vi "Calc dependand variables.vi"(11 "Item Names":string[][](array[string])) -> (3 "Dependand Variables":T1)   [LabVIEW 2025]
uses:
  Controls/Dependand_Variables.ctl
  <vilib>/Analysis/baseanly.llb/Mean (DBL).vi
  <vilib>/regexp/Match Regular Expression.xnode
  <vilib>/Analysis/NI_AALBase.lvlib
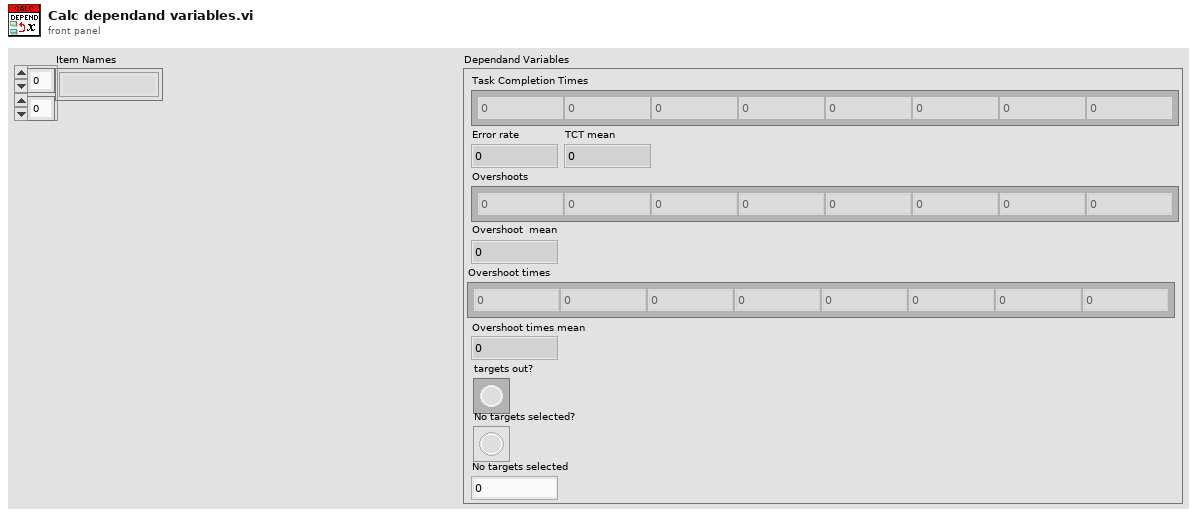
[diagram p1: front panel]
types:
  T1 = typedef "Dependand_Variables.ctl" = cluster{"Task Completion Times":dbl[], "TCT mean":dbl, "Error rate":i32, "Overshoots":i32[], "Overshoot  mean":dbl, "Overshoot times":dbl[], "Overshoot times mean":dbl, "targets out?":bool[], "No targets selected?":bool[], "No targets selected":i32}
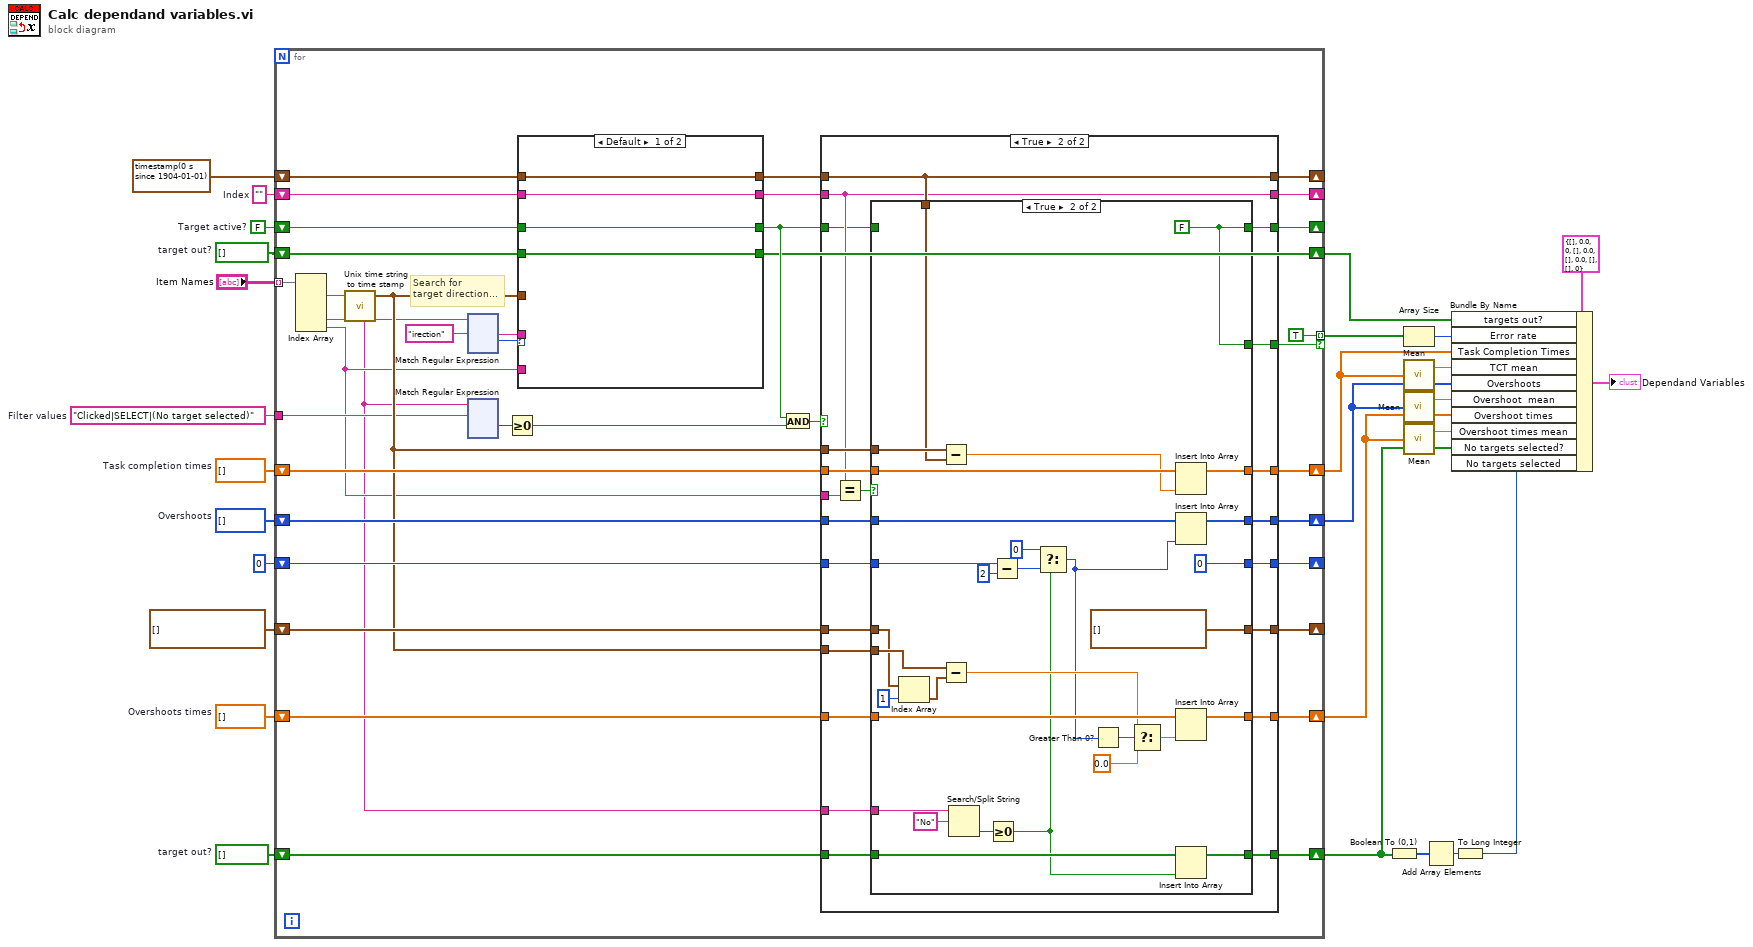
[diagram p0: block diagram]
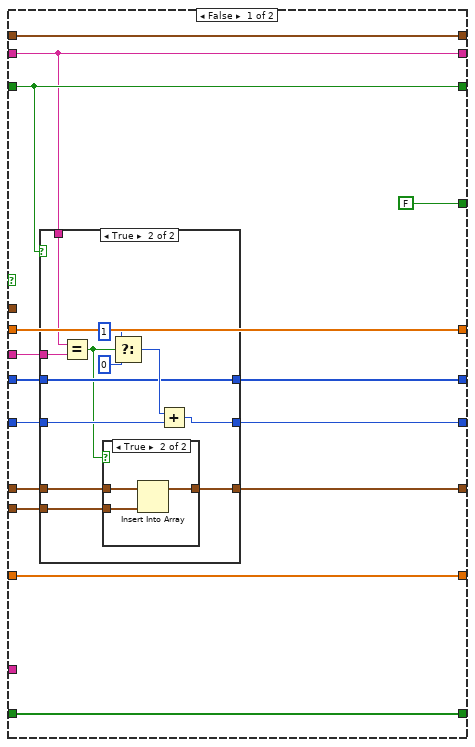
[diagram p2: hidden frame]
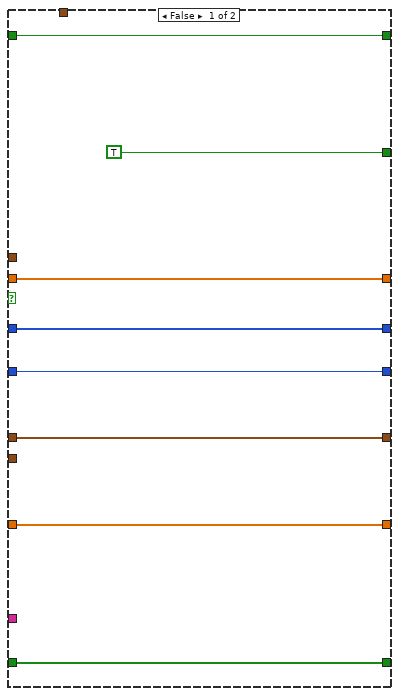
[diagram p5: hidden frame]
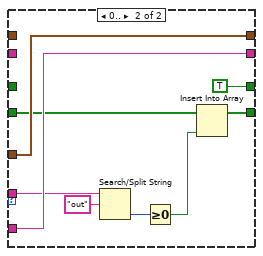
[diagram p6: hidden frame]
diagram:
  w5 = bool[] []  # target out?
  w7 = bool[] []  # target out?
  w18 = "Clicked|SELECT|(No target selected)"  # Filter values
  w27 = dbl[] []  # Overshoots times
  w24 = i32[] []  # Overshoots
  w23 = dbl[] []  # Task completion times
  w22 = FALSE  # Target active?
  w21 = ""  # Index
  n1 = for {
    tunnel: "Item Names" -> [w64] mode=indexing
    shift-right: [w57] -> _
    shift-left: timestamp(0 s since 1904-01-01) ("Time stamp") -> [w61]
    shift-right: [w56] -> _
    shift-left: w21 -> [w60]
    shift-right: [w54] -> _
    shift-left: w22 -> [w59]
    shift-right: [w52] -> w13
    shift-left: w23 -> [w53]
    tunnel: [TRUE] -> w16 mode=indexing if=w48
    shift-right: [w45] -> w11
    shift-left: w24 -> [w46]
    shift-right: [w43] -> _
    shift-left: 0 -> [w44]
    shift-right: [w40] -> _
    shift-left: timestamp[] [] -> [w42]
    shift-right: [w38] -> w9
    shift-left: w27 -> [w39]
    tunnel: w18 -> [w37]
    shift-right: [w34] -> w6
    shift-left: w7 -> [w33]
    shift-right: [w30] -> w4
    shift-left: w5 -> [w31]
    # "Search for\ntarget direction..."
    n2 = Index Array(array=w64) -> (element #1=w63:string, element #4=w28:string, element #5=w29:string)  [unwired: 5 in, 2 out]
    n3 = call "Unix time string to time stamp.vi"("Unix time string [ms]"=w63) -> ("Time stamp"=w41:timestamp)  [unwired: 4 in]
    n4 = xnode "Match Regular Expression"("input string"=w28, "regular expression"="irection" ("search string/char (-)")) -> ("after match"=w35:string, "offset past match"=w62:i32)  [unwired: 4 in, 3 out]
    n5 = xnode "Match Regular Expression"("input string"=w28, "regular expression"=w37) -> ("offset past match"=w47:i32)  [unwired: 4 in, 4 out]
    n6 = Greater Or Equal To 0?(x=w47) -> (x >= 0?=w32:bool)
    n7 = case shown="Default" w62 {
      tunnel: w41 -> [_ w406]
      tunnel: [w397 w406] -> w58
      tunnel: w61 -> [w397 _]
      tunnel: w29 -> [_ w405]
      tunnel: [w396 w405] -> w55
      tunnel: w60 -> [w396 _]
      tunnel: w59 -> [w395 _]
      tunnel: [w395 TRUE] -> w50
      tunnel: w35 -> [_ w403]
      tunnel: [w394 w399] -> w34
      tunnel: w33 -> [w394 w400]
      frame Default {
      }
      frame 0.. {
        n8 = Search/Split String(string=w403, search string/char (-)="out") -> (offset of match=w401:i32)  [unwired: 1 in, 2 out]
        n9 = Greater Or Equal To 0?(x=w401) -> (x >= 0?=w398:bool)
        n10 = Insert Into Array(array=w400, new element=w398) -> (w399:bool[])  [unwired: 1 in]
      }
    }
    n11 = And(x=w50, y=w32) -> (x .and. y?=w51:bool)
    n12 = case shown="True" w51 {
      tunnel: w41 -> [_ w353]
      tunnel: w58 -> [w313 w352]
      tunnel: [w313 w352] -> w57
      tunnel: [w308 w348] -> w56
      tunnel: w55 -> [w308 w348]
      tunnel: w50 -> [w310 w346]
      tunnel: [w310 w354] -> w54
      tunnel: w53 -> [w312 w351]
      tunnel: [w312 w350] -> w52
      tunnel: w29 -> [w309 w349]
      tunnel: [FALSE w345] -> w48
      tunnel: w46 -> [w304 w344]
      tunnel: [w305 w343] -> w45
      tunnel: w44 -> [w307 w342]
      tunnel: [w306 w341] -> w43
      tunnel: w42 -> [w303 w340]
      tunnel: w41 -> [w302 w338]
      tunnel: [w301 w339] -> w40
      tunnel: [w300 w337] -> w38
      tunnel: w39 -> [w300 w336]
      tunnel: w31 -> [w299 w335]
      tunnel: [w299 w334] -> w30
      tunnel: w28 -> [_ w333]
      frame False {
        n13 = case shown="True" w310 {
          tunnel: w309 -> [_ w328]
          tunnel: w308 -> [_ w327]
          tunnel: w307 -> [w316 w324]
          tunnel: [w316 w322] -> w306
          tunnel: [w315 w321] -> w305
          tunnel: w304 -> [w315 w321]
          tunnel: w303 -> [w314 w319]
          tunnel: w302 -> [_ w318]
          tunnel: [w314 w317] -> w301
          frame False {
          }
          frame True {
            n14 = Equal?(x=w327, y=w328) -> (x = y?=w320:bool)
            n15 = case shown="True" w320 {
              tunnel: w319 -> [w329 w332]
              tunnel: w318 -> [_ w331]
              tunnel: [w329 w330] -> w317
              frame False {
              }
              frame True {
                n16 = Insert Into Array(array=w332, new element=w331) -> (w330:timestamp[])  [unwired: 1 in]
              }
            }
            n17 = Select(t=1, s=w320, f=0 ("t")) -> (s? t:f=w323:i32)
            n18 = Add(x=w323, y=w324) -> (x+y=w322:i32)
          }
        }
      }
      frame True {
        n19 = Equal?(x=w348, y=w349) -> (x = y?=w347:bool)
        n20 = case shown="True" w347 {
          tunnel: [w362 w388] -> w354
          tunnel: w353 -> [_ w393]
          tunnel: w352 -> [_ w392]
          tunnel: w351 -> [w361 w391]
          tunnel: [w361 w389] -> w350
          tunnel: w346 -> [w362 _]
          tunnel: [TRUE w388] -> w345
          tunnel: w344 -> [w359 w387]
          tunnel: [w359 w386] -> w343
          tunnel: w342 -> [w358 w384]
          tunnel: [w358 0] -> w341
          tunnel: w340 -> [w356 w380]
          tunnel: [w356 timestamp[] []] -> w339
          tunnel: w338 -> [_ w381]
          tunnel: [w357 w377] -> w337
          tunnel: w336 -> [w357 w378]
          tunnel: w335 -> [w355 w371]
          tunnel: [w355 w370] -> w334
          tunnel: w333 -> [_ w367]
          frame False {
          }
          frame True {
            w388 = FALSE
            n21 = Index Array(array=w380, index=1) -> (element=w379:timestamp)
            n22 = Subtract(x=w393, y=w392) -> (x-y=w390:dbl)
            n23 = Subtract(x=w381, y=w379) -> (x-y=w374:dbl)
            n24 = Search/Split String(string=w367, search string/char (-)="No") -> (offset of match=w369:i32)  [unwired: 1 in, 2 out]
            n25 = Greater Or Equal To 0?(x=w369) -> (x >= 0?=w363:bool)
            n26 = Subtract(x=w384, y=2) -> (x-y=w366:i32)
            n27 = Select(t=0, s=w363, f=w366) -> (s? t:f=w365:i32)
            n28 = Greater Than 0?(x=w365) -> (x > 0?=w375:bool)
            n29 = Select(t=w374, s=w375, f=0.0) -> (s? t:f=w373:dbl)
            n30 = Insert Into Array(array=w391, new element=w390) -> (w389:dbl[])  [unwired: 1 in]
            n31 = Insert Into Array(array=w387, new element=w365) -> (w386:i32[])  [unwired: 1 in]
            n32 = Insert Into Array(array=w378, new element=w373) -> (w377:dbl[])  [unwired: 1 in]
            n33 = Insert Into Array(array=w371, new element=w363) -> (w370:bool[])  [unwired: 1 in]
          }
        }
      }
    }
  }
  n34 = Boolean To (0,1)(Boolean=w4) -> (0, 1=w3:i16[])
  n35 = Array Size(array=w16) -> (size(s)=w15:i32)
  n36 = call-poly <vilib>:"Mean.vi"("X"=w13) -> ("mean"=w14:dbl)  [unwired: 1 out]
  n37 = call-poly <vilib>:"Mean.vi"("X"=w11) -> ("mean"=w12:dbl)  [unwired: 1 out]
  n38 = call-poly <vilib>:"Mean.vi"("X"=w9) -> ("mean"=w10:dbl)  [unwired: 1 out]
  n39 = Add Array Elements(numeric array=w3) -> (sum=w2:i16)
  n40 = To Long Integer(number=w2) -> (32bit integer=w1:i32)
  n41 = Bundle By Name(cluster=T1 {"Task Completion Times"=[], "TCT mean"=0.0, "Error rate"=0, "Overshoots"=[], "Overshoot  mean"=0.0, "Overshoot times"=[], "Overshoot times mean"=0.0, "targets out?"=[], "No targets selected?"=[], "No targets selected"=0} ("Cluster"), "targets out?"=w6, "Error rate"=w15, "Task Completion Times"=w13, "TCT mean"=w14, "Overshoots"=w11, "Overshoot  mean"=w12, "Overshoot times"=w9, "Overshoot times mean"=w10, "No targets selected?"=w4, "No targets selected"=w1) -> (→"Dependand Variables":T1)
